vi "Database Fetching.vi"() -> ()   [LabVIEW 2013]
doc: "This example fetches data from the specified table in a database named LabVIEW.mdb located in the LabVIEW examples>>database directory.\n\nThe table is assumed to be in the same format with the same datatypes as defined by the fetchdata table. You can use the Next and Previous buttons to move from the current record in the database table to the next or previous record."
uses:
  Auxilliary.llb/DB Tools Cursor Type.ctl
  Connection.llb/DB Tools Open Connec (Path).vi
  Connection.llb/Conn Execute.vi
  Recordset.llb/Rec Get Recordset Properties (R).vi
  Recordset.llb/Rec Destroy - Connection.vi
  Recordset.llb/Rec Move To Previous Record (R).vi
  Recordset.llb/Rec Move To Next Record (R).vi
  Recordset.llb/Rec Fetch Integer Data (R).vi
  Recordset.llb/Rec Fetch String Data (R).vi
  Recordset.llb/Rec Fetch Binary Data (R).vi
  _DB Variant To Data/Database Variant To Data.xnode
  NI_Database_API_64.lvlib
panel:
  in  "table":enum16{"fetchdata", "fetchempty"}(ring)
  out "record number":i32
  in  "stop":bool
  out "Phone Number":string
  out "Customer Number":i32
  out "Last Name":string
  out "First Name":string
  in  "previous record":bool
  in  "next record":bool
  # "INSTRUCTIONS:\n\nChoose the table from which to select data.  Run the VI.  Use the next record and previous record buttons to navigate the recordset. Press stop when finished."
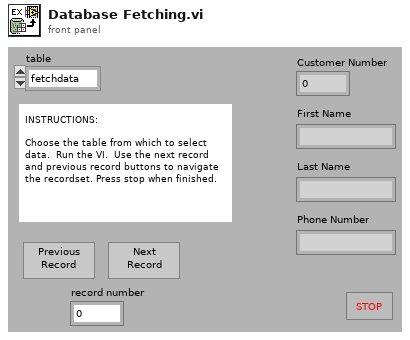
[diagram p1: front panel]
types:
  T1 = typedef "NI_Database_API_64.lvlib/DB Tools Cursor Type.ctl" = enum16{"forward-only", "keyset", "dynamic", "static"}
  T2 = typedef "NI_Database_API_64.lvlib/Conn ObjectReference.ctl" = refnum<k1>
  T3 = typedef "NI_Database_API_64.lvlib/Rec ObjectReference.ctl" = refnum<k1>
  T4 = typedef "NI_Database_API_64.lvlib/Rec Properties.ctl" = cluster{"column count":i32, "record index":i32, "record count":i32, "bof?":bool, "eof?":bool, "cursor type":T1, "cache size":i32, "state":enum16{"closed", "open"}}
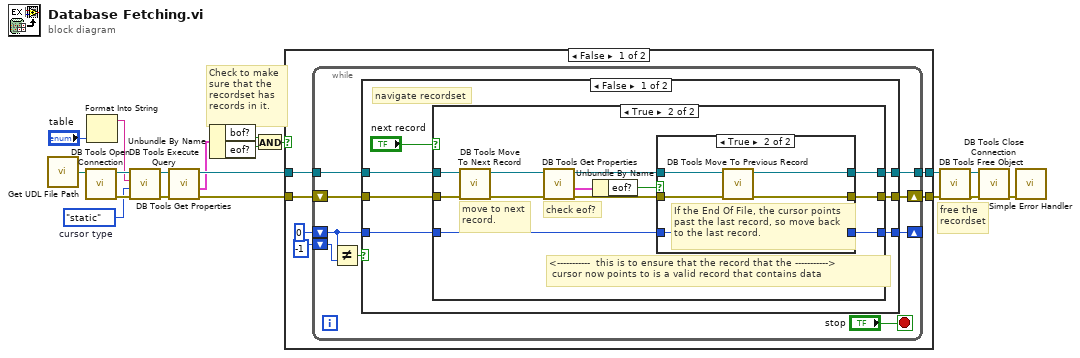
[diagram p0: block diagram]
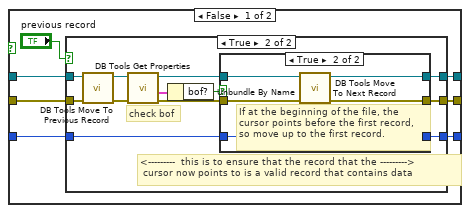
[diagram p2: hidden frame]
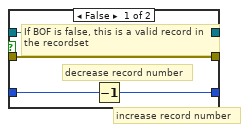
[diagram p4: hidden frame]
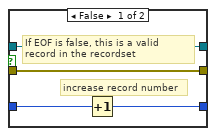
[diagram p5: hidden frame]
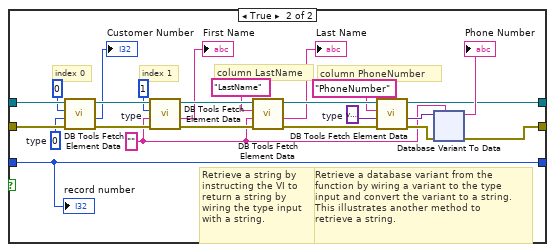
[diagram p6: hidden frame]
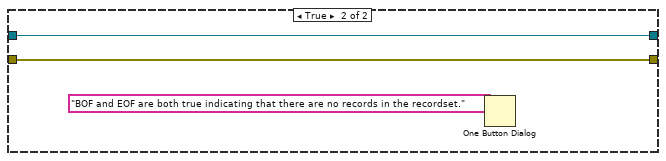
[diagram p7: hidden frame]
diagram:
  w16 = DB_Tools_Cursor_Type."static"  # cursor type
  # "free the\nrecordset"
  # "Check to make\nsure that the\nrecordset has\nrecords in it."
  n1 = call "Get UDL File Path.vi"() -> ("UDL file path"=w19:path)  [unwired: 1 in]
  n2 = call-poly "DB Tools Open Connection.vi"("connection information"=w19) -> ("error out"=w18:errorcluster, "connection reference"=w17:T2)  [unwired: 7 in]
  n3 = Format Into String("table") -> (resulting string=w2:string)  [unwired: 3 in, 1 out]
  n4 = call-poly "DB Tools Execute Query.vi"("error in (no error)"=w18, "cursor type"=w16, "SQL query"=w2, "connection reference"=w17) -> ("error out"=w14:errorcluster, "recordset reference"=w15:T3)  [unwired: 4 in]
  n5 = call-poly "DB Tools Get Properties.vi"("error in (no error)"=w14, "recordset reference"=w15) -> ("error out"=w12:errorcluster, "recordset properties"=w11:T4, "recordset reference out"=w13:T3)  [unwired: 3 in]
  n6 = Unbundle By Name(w11) -> ("bof?"=w9:bool, "eof?"=w8:bool)
  n7 = And(x=w9, y=w8) -> (x .and. y?=w10:bool)
  n8 = case shown="False" w10 {
    tunnel: w13 -> [w25 w152]
    tunnel: w12 -> [w22 w151]
    tunnel: [w21 w152] -> w6
    tunnel: [w20 w151] -> w7
    frame False {
      n9 = while {
        tunnel: w25 -> [w34]
        shift-right: [w29] -> _
        shift-left: 0 -> [w31]
        shift-left: -1 -> [w32]
        shift-right: [w28] -> w20
        shift-left: w22 -> [w27]
        tunnel: [w26] -> w21
        stop <- "stop" stop-if-true
        n10 = Not Equal?(x=w31, y=w32) -> (x != y?=w30:bool)
        n11 = case shown="False" w30 {
          tunnel: w27 -> [w40 w117]
          tunnel: w34 -> [w39 w116]
          tunnel: w31 -> [w38 w97]
          tunnel: [w37 w97] -> w29
          tunnel: [w36 w95] -> w28
          tunnel: [w35 w96] -> w26
          frame False {
            # "navigate recordset"
            n12 = case shown="True" "next record" {
              tunnel: w38 -> [w48 w80]
              tunnel: [w47 w79] -> w37
              tunnel: w40 -> [w45 w74]
              tunnel: [w46 w78] -> w36
              tunnel: w39 -> [w44 w75]
              tunnel: [w42 w73] -> w35
              frame False {
                n13 = case shown="True" "previous record" {
                  tunnel: w48 -> [w51 w55]
                  tunnel: [w51 w53] -> w47
                  tunnel: w45 -> [w50 w62]
                  tunnel: w44 -> [w49 w63]
                  tunnel: [w50 w56] -> w46
                  tunnel: [w49 w52] -> w42
                  frame False {
                  }
                  frame True {
                    # "<---------  this is to ensure that the record that the --------->\n cursor now points to is a valid record that contains data"
                    # "check bof"
                    n14 = call-poly "DB Tools Move To Previous Record.vi"("error in (no error)"=w62, "recordset reference"=w63) -> ("error out"=w61:errorcluster, "recordset reference out"=w60:T3)  [unwired: 8 in]
                    n15 = call-poly "DB Tools Get Properties.vi"("error in (no error)"=w61, "recordset reference"=w60) -> ("error out"=w58:errorcluster, "recordset properties"=w59:T4, "recordset reference out"=w57:T3)  [unwired: 3 in]
                    n16 = Unbundle By Name(w59) -> ("bof?"=w54:bool)
                    n17 = case shown="True" w54 {
                      tunnel: w57 -> [w64 w72]
                      tunnel: w58 -> [w65 w71]
                      tunnel: w55 -> [w67 w70]
                      tunnel: [w66 w70] -> w53
                      tunnel: [w65 w69] -> w56
                      tunnel: [w64 w68] -> w52
                      frame False {
                        # "If BOF is false, this is a valid record in \nthe recordset"
                        # "decrease record number"
                        # "increase record number"
                        n18 = Decrement(x=w67) -> (x-1=w66:i32)
                      }
                      frame True {
                        # "If at the beginning of the file, the \ncursor points before the first record, \nso move up to the first record."
                        n19 = call-poly "DB Tools Move To Next Record.vi"("error in (no error)"=w71, "recordset reference"=w72) -> ("error out"=w69:errorcluster, "recordset reference out"=w68:T3)  [unwired: 8 in]
                      }
                    }
                  }
                }
              }
              frame True {
                # "<-----------  this is to ensure that the record that the ----------->\n cursor now points to is a valid record that contains data"
                # "check eof?"
                # "move to next\nrecord."
                n20 = call-poly "DB Tools Move To Next Record.vi"("error in (no error)"=w74, "recordset reference"=w75) -> ("error out"=w77:errorcluster, "recordset reference out"=w76:T3)  [unwired: 8 in]
                n21 = call-poly "DB Tools Get Properties.vi"("error in (no error)"=w77, "recordset reference"=w76) -> ("error out"=w81:errorcluster, "recordset properties"=w84:T4, "recordset reference out"=w82:T3)  [unwired: 3 in]
                n22 = Unbundle By Name(w84) -> ("eof?"=w83:bool)
                n23 = case shown="True" w83 {
                  tunnel: w82 -> [w85 w93]
                  tunnel: w81 -> [w86 w92]
                  tunnel: w80 -> [w88 w91]
                  tunnel: [w87 w91] -> w79
                  tunnel: [w86 w90] -> w78
                  tunnel: [w85 w89] -> w73
                  frame False {
                    # "If EOF is false, this is a valid record in the recordset"
                    # "increase record number"
                    n24 = Increment(x=w88) -> (x+1=w87:i32)
                  }
                  frame True {
                    # "If the End Of File, the cursor points\npast the last record, so move back \nto the last record."
                    n25 = call-poly "DB Tools Move To Previous Record.vi"("error in (no error)"=w92, "recordset reference"=w93) -> ("error out"=w90:errorcluster, "recordset reference out"=w89:T3)  [unwired: 8 in]
                  }
                }
              }
            }
          }
          frame True {
            w102 = 0  # type
            w105 = variant  # type
            w94 = ""  # type
            # "Retrieve a database variant from the\nfunction by wiring a variant to the type\ninput and convert the variant to a string.  \nThis illustrates another method to\nretrieve a string."
            # "Retrieve a string by \ninstructing the VI to \nreturn a string by \nwiring the type input \nwith a string."
            # "column PhoneNumber"
            # "column LastName"
            # "index 1"
            # "index 0"
            n26 = call-poly "DB Tools Fetch Element Data.vi"("error in (no error)"=w117, "type"=w102, "column index"=0, "recordset reference"=w116) -> ("error out"=w115:errorcluster, "data"=→"Customer Number":i32, "recordset reference out"=w114:T3)  [unwired: 3 in]
            n27 = call-poly "DB Tools Fetch Element Data.vi"("error in (no error)"=w115, "type"=w94, "column index"=1, "recordset reference"=w114) -> ("error out"=w113:errorcluster, "data"=→"First Name":string, "recordset reference out"=w112:T3)  [unwired: 3 in]
            n28 = call-poly "DB Tools Fetch Element Data.vi"("error in (no error)"=w113, "type"=w94, "column index"="LastName" ("SQL query"), "recordset reference"=w112) -> ("error out"=w111:errorcluster, "data"=→"Last Name":string, "recordset reference out"=w110:T3)  [unwired: 3 in]
            n29 = call-poly "DB Tools Fetch Element Data.vi"("error in (no error)"=w111, "type"=w105, "column index"="PhoneNumber" ("SQL query"), "recordset reference"=w110) -> ("error out"=w103:errorcluster, "data"=w104:variant, "recordset reference out"=w96:T3)  [unwired: 3 in]
            n30 = xnode "Database Variant To Data"("database variant"=w104, "error in"=w103, "type"=w94) -> ("data"=→"Phone Number":string, "error out"=w95:errorcluster)
            "record number" <- w97
          }
        }
      }
    }
    frame True {
      n31 = One Button Dialog(message="BOF and EOF are both true indicating that there are no records in the recordset.") -> ()  [unwired: 1 in, 1 out]
    }
  }
  n32 = call-poly "DB Tools Free Object.vi"("error in (no error)"=w7, "recordset reference"=w6) -> ("error out"=w4:errorcluster, "connection reference"=w5:T2)  [unwired: 8 in]
  n33 = call "DB Tools Close Connection.vi"("error in (no error)"=w4, "connection reference"=w5) -> ("error out"=w1:errorcluster)  [unwired: 5 in]
  n34 = call <vilib>:"Simple Error Handler.vi"("error in (no error)"=w1) -> ()  [unwired: 4 in, 5 out]
